vi "generate target 1.vi"(4 "PICTURE SIZE Y":dbl, 6 "PICTURE SIZE X":dbl, 8 "number of targets":i32, 10 "spacing limit":i32) -> (2 "Array 2":cluster{"Numeric":i32, "Numeric 2":i32}[](array[cluster]))   [LabVIEW 2014]
panel:
  in  "Array":cluster{"Numeric":i32, "Numeric 2":i32}[](array[cluster])
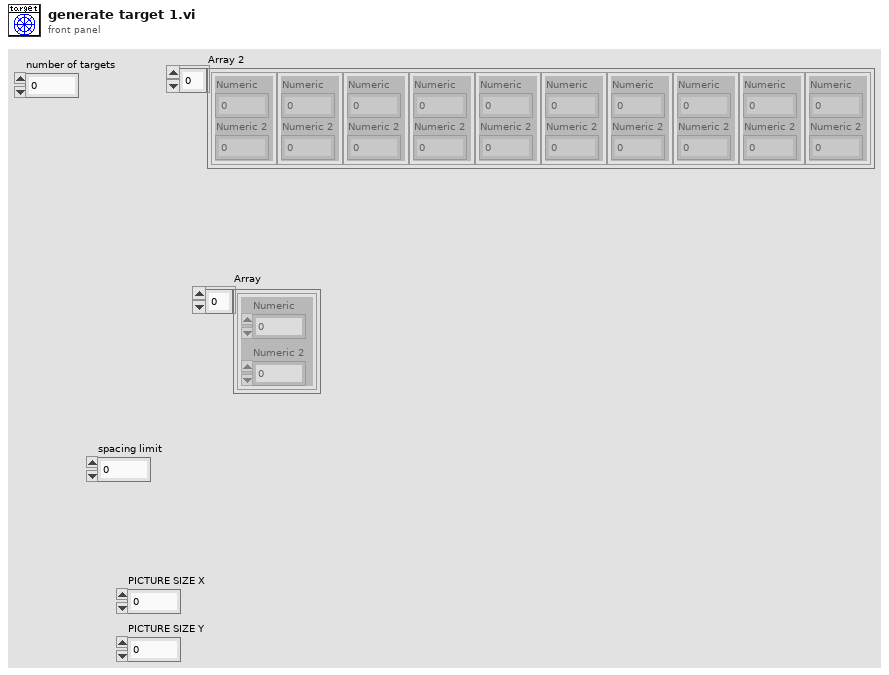
[diagram p1: front panel]
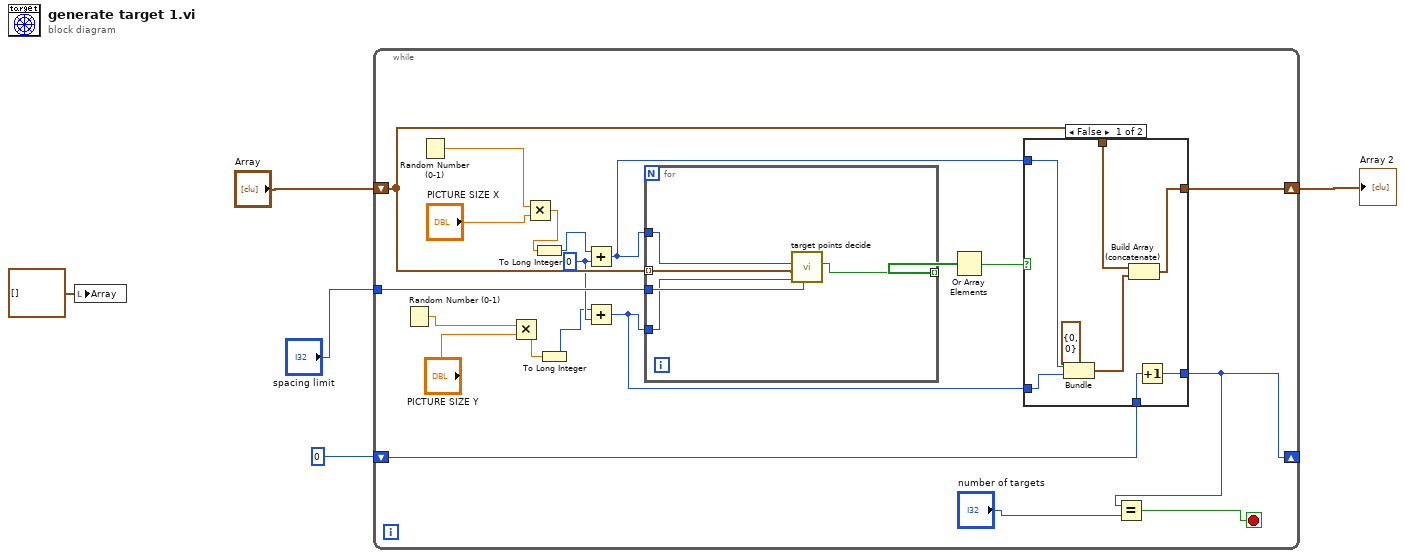
[diagram p0: block diagram]
diagram:
  n1 = local write "Array"(cluster{"Numeric":i32, "Numeric 2":i32}[] [] ("Array")) -> ()
  n2 = while {
    shift-right: [w16] -> w2
    shift-left: "Array" -> [w17]
    tunnel: "spacing limit" -> [w10]
    shift-right: [w12] -> _
    shift-left: 0 -> [w13]
    stop <- w15 stop-if-true
    w9 = 0 ("y")
    n3 = Random Number (0-1)() -> (number: 0 to 1=w22:dbl)
    n4 = Random Number (0-1)() -> (number: 0 to 1=w21:dbl)
    n5 = Multiply(x=w22, y="PICTURE SIZE Y") -> (x*y=w19:dbl)
    n6 = Multiply(x=w21, y="PICTURE SIZE X") -> (x*y=w18:dbl)
    n7 = To Long Integer(number=w18) -> (32bit integer=w11:i32)
    n8 = To Long Integer(number=w19) -> (32bit integer=w8:i32)
    n9 = Add(x=w11, y=w9) -> (x+y=w6:i32)
    n10 = Add(x=w8, y=w9) -> (x+y=w7:i32)
    n11 = for {
      tunnel: w17 -> [w35] mode=indexing
      tunnel: w10 -> [w39]
      tunnel: [w38] -> w25 mode=indexing
      tunnel: w6 -> [w37]
      tunnel: w7 -> [w36]
      n12 = call "target points decide.vi"("Spacing limit"=w39, "Y"=w36, "Cluster"=w35, "X"=w37) -> ("too close?"=w38:bool)  [unwired: 7 in]
    }
    n13 = Or Array Elements(Boolean array=w25) -> (logical OR=w24:bool)
    n14 = case shown="False" w24 {
      tunnel: w6 -> [w32 _]
      tunnel: w7 -> [w31 _]
      tunnel: w17 -> [w29 w34]
      tunnel: [w28 w34] -> w16
      tunnel: w13 -> [w27 w33]
      tunnel: [w26 w33] -> w12
      frame False {
        (unwired) cluster{i32, i32} {0, 0} ("cluster")
        n15 = Bundle(w32, w31) -> (w30:cluster{i32, i32})  [unwired: 1 in]
        n16 = Build Array (concatenate)(w29, w30) -> (w28:cluster{"Numeric":i32, "Numeric 2":i32}[])
        n17 = Increment(x=w27) -> (x+1=w26:i32)
      }
      frame True {
      }
    }
    n18 = Equal?(x=w12, y="number of targets") -> (x = y?=w15:bool)
  }
  "Array 2" <- w2
